vi "Set Pattern.vi"(5 "Write to FPGA(T)":bool=TRUE, 7 "error in (no error)":errorcluster, 9 "IO Lines Patttern Settings":T1[](array[typedef]) {"Duration (us)" min=0.005 max=42550000.0 step=0.005 format="%#.3f"}, 10 "FPGA VI Reference In":refnum<k20>) -> (0 "error out":errorcluster, 2 "Pattern Digital Data":digitaldata, 3 "FPGA VI Reference Out":refnum<k20>)   [LabVIEW 2016]
uses:
  Typedefs/IO Lines State.ctl
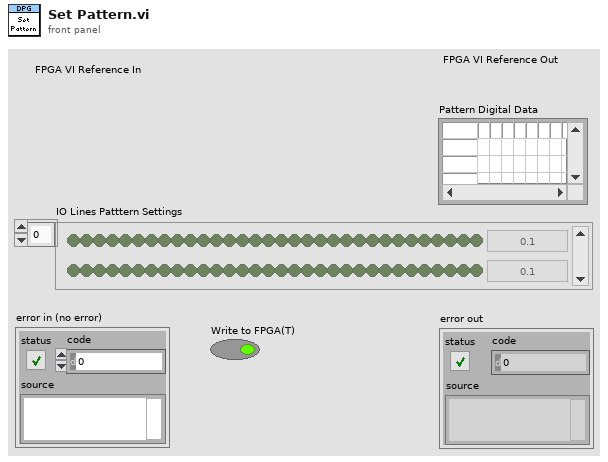
[diagram p1: front panel]
types:
  T1 = typedef "IO Lines State.ctl" = cluster{"State":bool[], "Duration (us)":dbl}
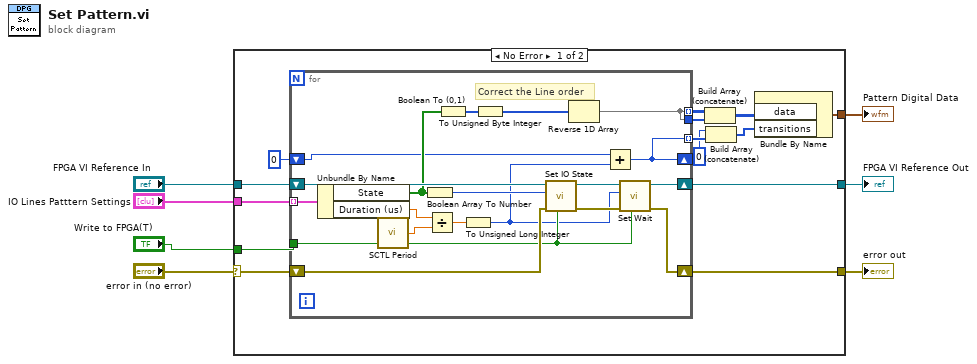
[diagram p0: block diagram]
diagram:
  n1 = case shown="No Error" "error in (no error)" {
    selector: "error in (no error)" -> [w20 w42]
    tunnel: [w18 w42] -> w6
    tunnel: "IO Lines Patttern Settings" -> [w21 _]
    tunnel: "FPGA VI Reference In" -> [w19 w41]
    tunnel: "Write to FPGA(T)" -> [w17 _]
    tunnel: [w13 _] -> w2
    tunnel: [w12 w41] -> w1
    frame No Error {
      n2 = for {
        tunnel: w21 -> [w40] mode=indexing
        shift-right: [w32] -> w18
        shift-left: w20 -> [w35]
        tunnel: w17 -> [w31]
        tunnel: [w22] -> w15 mode=indexing
        tunnel: [w26] -> w14 mode=indexing
        shift-right: [w26] -> _
        shift-left: u32 0 -> [w27]
        shift-right: [w23] -> w12
        shift-left: w19 -> [w33]
        tunnel: [w22] -> w10
        # "Correct the Line order"
        n3 = Unbundle By Name(w40) -> ("State"=w30:bool[], "Duration (us)"=w39:dbl)
        n4 = call "SCTL Period.vi"() -> ("Clock Period(micro second)"=w38:dbl)  [unwired: 15 in]
        n5 = Boolean Array To Number(Boolean array=w30) -> (number=w37:u32)
        n6 = Divide(x=w39, y=w38) -> (x/y=w36:dbl)
        n7 = Boolean To (0,1)(Boolean=w30) -> (0, 1=w29:i16[])
        n8 = To Unsigned Long Integer(number=w36) -> (unsigned 32bit integer=w28:u32)
        n9 = To Unsigned Byte Integer(number=w29) -> (unsigned 8bit integer=w25:u8[])
        n10 = call "Set IO State.vi"("Write to FPGA(T)"=w31, "error in (no error)"=w35, "IO State"=w37, "FPGA VI Reference In"=w33) -> ("error out"=w34:errorcluster, "FPGA VI Reference Out"=w24:refnum<k20>)  [unwired: 6 in]
        n11 = Reverse 1D Array(array=w25) -> (reversed array=w22:u8[])
        n12 = Add(x=w27, y=w28) -> (x+y=w26:u32)
        n13 = call "Set Wait.vi"("Write to FPGA(T)"=w31, "error in (no error)"=w34, "Duration"=w28, "FPGA VI Reference In"=w24) -> ("error out"=w32:errorcluster, "FPGA VI Reference Out"=w23:refnum<k20>)  [unwired: 6 in]
      }
      n14 = Build Array (concatenate)(w15, w10) -> (w11:u8[][])
      n15 = Build Array (concatenate)(u32 0, w14) -> (w9:u32[])
      n16 = Bundle By Name("data"=w11, "transitions"=w9) -> (w13:digitaldata)  [unwired: 1 in]
    }
    frame Error {
    }
  }
  "error out" <- w6
  "Pattern Digital Data" <- w2
  "FPGA VI Reference Out" <- w1
